vi "FGV - Attocube Remote.vi"(4 "error in":errorcluster, 6 "Function":enum16{"write", "read"}(ring), 7 "Attocube Remote":bool) -> (0 "error out":errorcluster, 3 "Attocube Remote":bool)   [LabVIEW 2013]
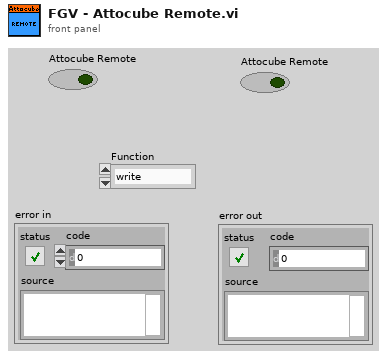
[diagram p1: front panel]
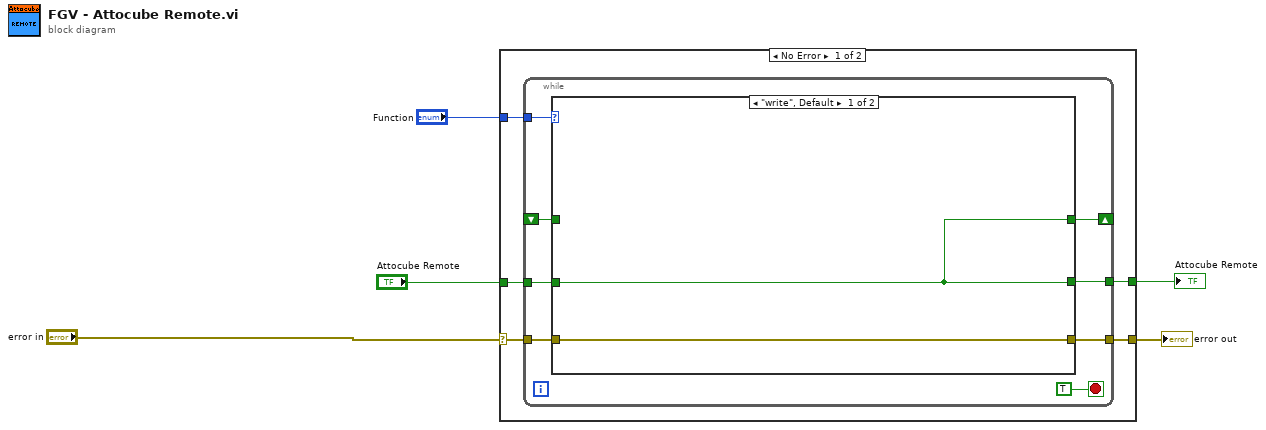
[diagram p0: block diagram]
diagram:
  n1 = case shown="No Error" "error in" {
    selector: "error in" -> [w10 w24]
    tunnel: [w6 w24] -> w5
    tunnel: [w9 w23] -> w2
    tunnel: "Function" -> [w8 _]
    tunnel: "Attocube Remote" -> [w7 w23]
    frame No Error {
      n2 = while {
        shift-right: [w14] -> _
        shift-left: _ -> [w13]
        tunnel: w10 -> [w17]
        tunnel: [w16] -> w9
        tunnel: w8 -> [w15]
        tunnel: w7 -> [w12]
        tunnel: [w11] -> w6
        stop <- TRUE stop-if-true
        n3 = case shown="\"write\", Default" w15 {
          tunnel: w17 -> [w19 w21]
          tunnel: [w20 w22] -> w16
          tunnel: [w20 w22] -> w14
          tunnel: w13 -> [_ w22]
          tunnel: w12 -> [w20 _]
          tunnel: [w19 w21] -> w11
          frame "write", Default {
          }
          frame "read" {
          }
        }
      }
    }
    frame Error {
    }
  }
  "error out" <- w5
  "Attocube Remote" <- w2
